vi "CalMic-Load Calibration Log.vi"(0 "Cal Log":path) -> (4 "Array":string[][](array[string]), 8 "Last":dbl)   [LabVIEW 2020]
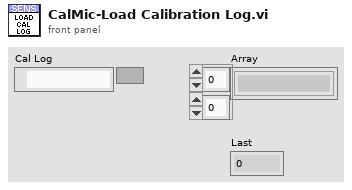
[diagram p1: front panel]
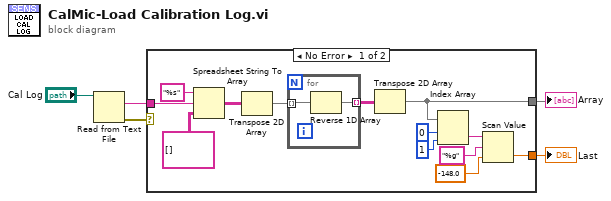
[diagram p0: block diagram]
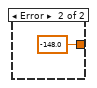
[diagram p2: hidden frame]
diagram:
  n1 = Read from Text File(file (use dialog)="Cal Log") -> (text=w2:string, error out=w3:errorcluster)  [unwired: 3 in, 2 out]
  n2 = case shown="No Error" w3 {
    tunnel: w2 -> [w18 _]
    tunnel: [w12 _] -> w5
    tunnel: [w8 -148.0] -> w1
    frame No Error {
      n3 = Spreadsheet String To Array(format string="%s", spreadsheet string=w18, array type (2D Dbl)=string[][] []) -> (array=w15:string[][])  [unwired: 1 in]
      n4 = Transpose 2D Array(2D array=w15) -> (transposed array=w14:string[][])
      n5 = for {
        tunnel: w14 -> [w20] mode=indexing
        tunnel: [w19] -> w13 mode=indexing
        n6 = Reverse 1D Array(array=w20) -> (reversed array=w19:string[])
      }
      n7 = Transpose 2D Array(2D array=w13) -> (transposed array=w12:string[][])
      n8 = Index Array(array=w12, index (row)=0, index (col)=1 ("disabled index (col)")) -> (element=w9:string)
      n9 = Scan Value(string=w9, format string="%g", default (0 dbl)=-148.0) -> (value=w8:dbl)  [unwired: 1 out]
    }
    frame Error {
    }
  }
  "Array" <- w5
  "Last" <- w1
